vi "Extract Latest.vi"(8 "Error":errorcluster, 10 "Raw Data Waveform":T1, 11 "(Index_Pointer)":refnum<class "Index_Pointer.lvclass">) -> (0 "Error Out":errorcluster, 2 "Waveform Out":T1, 3 "(Index_Pointer) Out":refnum<class "Index_Pointer.lvclass">)   [LabVIEW 2024, in "Index_Pointer.lvclass"]
uses:
  Index_Pointer.lvclass
  Universal Controls/Waveform_Data.ctl
  Index_Pointer.lvclass/Index_Pointer.ctl
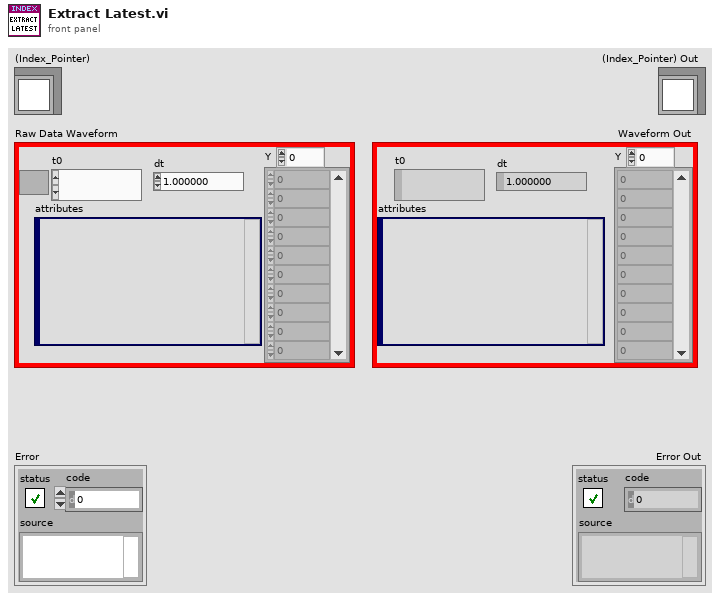
[diagram p1: front panel]
types:
  T1 = typedef "Waveform_Data.ctl" = waveform(dbl)
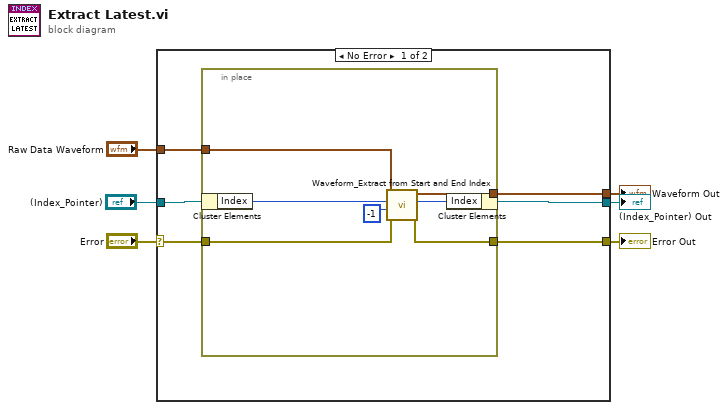
[diagram p0: block diagram]
diagram:
  n1 = case shown="No Error" "Error" {
    selector: "Error" -> [w12 w21]
    tunnel: [w11 w21] -> w5
    tunnel: "Raw Data Waveform" -> [w7 _]
    tunnel: "(Index_Pointer)" -> [w9 w20]
    tunnel: [w8 w20] -> w2
    tunnel: [w10 _] -> w1
    frame No Error {
      n2 = in-place {
        in-place-border: w12 -> [w19]
        in-place-border: [w18] -> w11
        in-place-border: [w16] -> w10
        in-place-border: w7 -> [w13]
        n3 = in-place-cluster #1(w9) -> ("Index"=w15:i32)
        n4 = call "Waveform_Extract from Start and End Index.vi"("Error"=w19, "End Index\n(-1) Last point"=-1 ("End Index\n(-1) Last point"), "Start Index"=w15, "Raw Data Waveform"=w13) -> ("Error Out"=w18:errorcluster, "Start Out"=w14:i32, "Waveform Out"=w16:T1)  [unwired: 5 out]
        n5 = in-place-cluster #1("Index"=w14) -> (w8:refnum<class "Index_Pointer.lvclass">)
      }
    }
    frame Error {
    }
  }
  "Error Out" <- w5
  "(Index_Pointer) Out" <- w2
  "Waveform Out" <- w1
